vi "CODMn插入数据.vi"(1 "data":T3 {"单位" items=["ug/L", "mg/L", "ppm", "mg/m3", "cm", "ppb", "ug/m3", "%", "nmol/mol", "umol/mol", "MPN/L", "MPN/100ml", "ng/m3", "NTU", "无量纲", "ms/cm", "us/cm"]}, 2 "CODMn关键参数":T2, 3 "SN":string, 5 "table":string, 7 "测量模式":T4(ring)=enum."水样测试", 9 "数据类型":string(combo)="N", 11 "error in (no error)":errorcluster) -> (15 "error out":errorcluster)   [LabVIEW 2016, in "斯坦道CODMn新电路板.lvlib"]
uses:
  <vilib>/Utility/error.llb/DialogType.ctl
panel:
  in  "data 2":T1={"时间"=timestamp(0 s since 1904-01-01), "测量模式"="水样测试", "数据类型"="N", "检测值"=0.0, "单位"="mg/L", "数据标识"="N", "终点滴定数"=0.0, "量程"=0.0, "SN"="", "标样参考值"=0.0, "跨度值"=0.0, "A"=0, "B"=0, "K"=0, "环境温度"=0.0, "加热实时温度"=0.0, "因子编码"="", "X0"=0.0, "X^2"=0.0, "X"=0.0, "B 2"=0.0, "光值1"=0.0, "光值2"=0.0, "光值3"=0.0, "光值4"=0.0, "光值5"=0.0, "光值6"=0.0, "光值7"=0.0, "光值8"=0.0, "测量量程"=0.0, "测量检出限"=0.0, "测量精度"=0.0, "测量间隔"=0.0, "消解温度"=0.0, "消解时长"=0.0, "三项式系数"=0.0, "二次多项式系数"=0.0, "曲线斜率"=0.0, "曲线截距"=0.0, "线性相关系数"=0.0, "空白校准时间"=timestamp(0 s since 1904-01-01), "标样校准时间"=timestamp(0 s since 1904-01-01), "测量信号值"=0.0, "稀释倍数"=0.0, "量程系数"=0.0, "LastTime"=timestamp(0 s since 1904-01-01)}
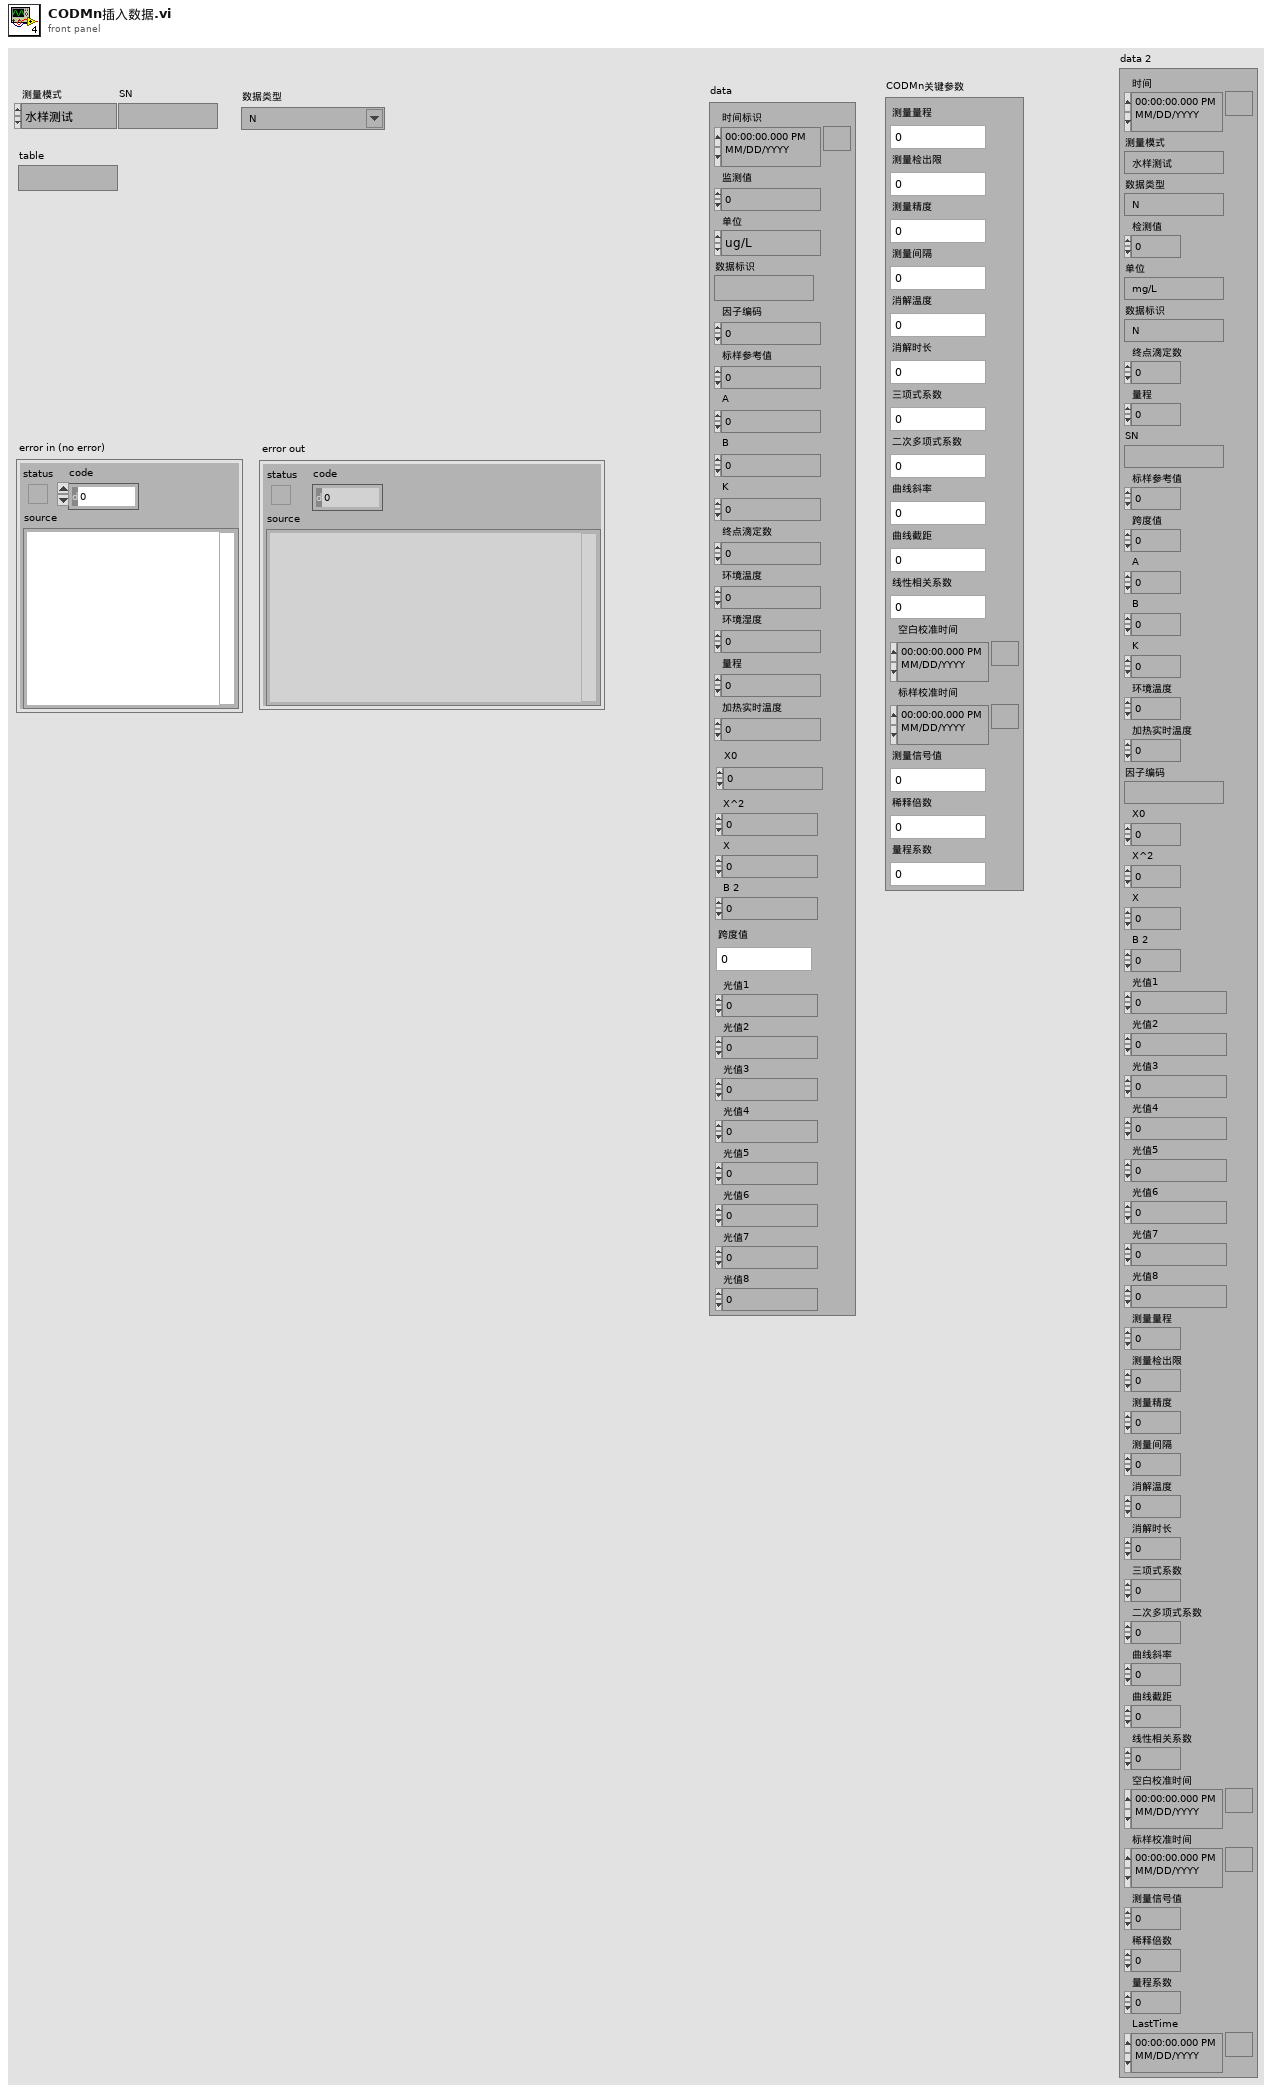
[diagram p1: front panel]
types:
  T1 = cluster{"时间":timestamp, "测量模式":string, "数据类型":string, "检测值":sgl, "单位":string, "数据标识":string, "终点滴定数":sgl, "量程":sgl, "SN":string, "标样参考值":sgl, "跨度值":sgl, "A":u32, "B":u32, "K":u32, "环境温度":sgl, "加热实时温度":sgl, "因子编码":string, "X0":sgl, "X^2":sgl, "X":sgl, "B 2":sgl, "光值1":sgl, "光值2":sgl, "光值3":sgl, "光值4":sgl, "光值5":sgl, "光值6":sgl, "光值7":sgl, "光值8":sgl, "测量量程":sgl, "测量检出限":sgl, "测量精度":sgl, "测量间隔":sgl, "消解温度":sgl, "消解时长":sgl, "三项式系数":sgl, "二次多项式系数":sgl, "曲线斜率":sgl, "曲线截距":sgl, "线性相关系数":sgl, "空白校准时间":timestamp, "标样校准时间":timestamp, "测量信号值":sgl, "稀释倍数":sgl, "量程系数":sgl, "LastTime":timestamp}
  T2 = cluster{"测量量程":sgl, "测量检出限":sgl, "测量精度":sgl, "测量间隔":sgl, "消解温度":sgl, "消解时长":sgl, "三项式系数":sgl, "二次多项式系数":sgl, "曲线斜率":sgl, "曲线截距":sgl, "线性相关系数":sgl, "空白校准时间":timestamp, "标样校准时间":timestamp, "测量信号值":sgl, "稀释倍数":sgl, "量程系数":sgl}
  T3 = cluster{"时间标识":timestamp, "监测值":sgl, "单位":u16, "数据标识":string, "因子编码":u32, "标样参考值":sgl, "A":sgl, "B":sgl, "K":sgl, "终点滴定数":sgl, "环境温度":sgl, "环境湿度":sgl, "量程":sgl, "加热实时温度":sgl, "X0":sgl, "X^2":sgl, "X":sgl, "B 2":sgl, "跨度值":sgl, "光值1":sgl, "光值2":sgl, "光值3":sgl, "光值4":sgl, "光值5":sgl, "光值6":sgl, "光值7":sgl, "光值8":sgl}
  T4 = enum16{"维护数据", "水样测试", "标样核查", "零点核查", "跨度核查", "空白测试", "平行样测试", "加标回收", "空白校准", "标样校准", "初始化（清洗）"}
  T5 = typedef "DialogType.ctl" = u16
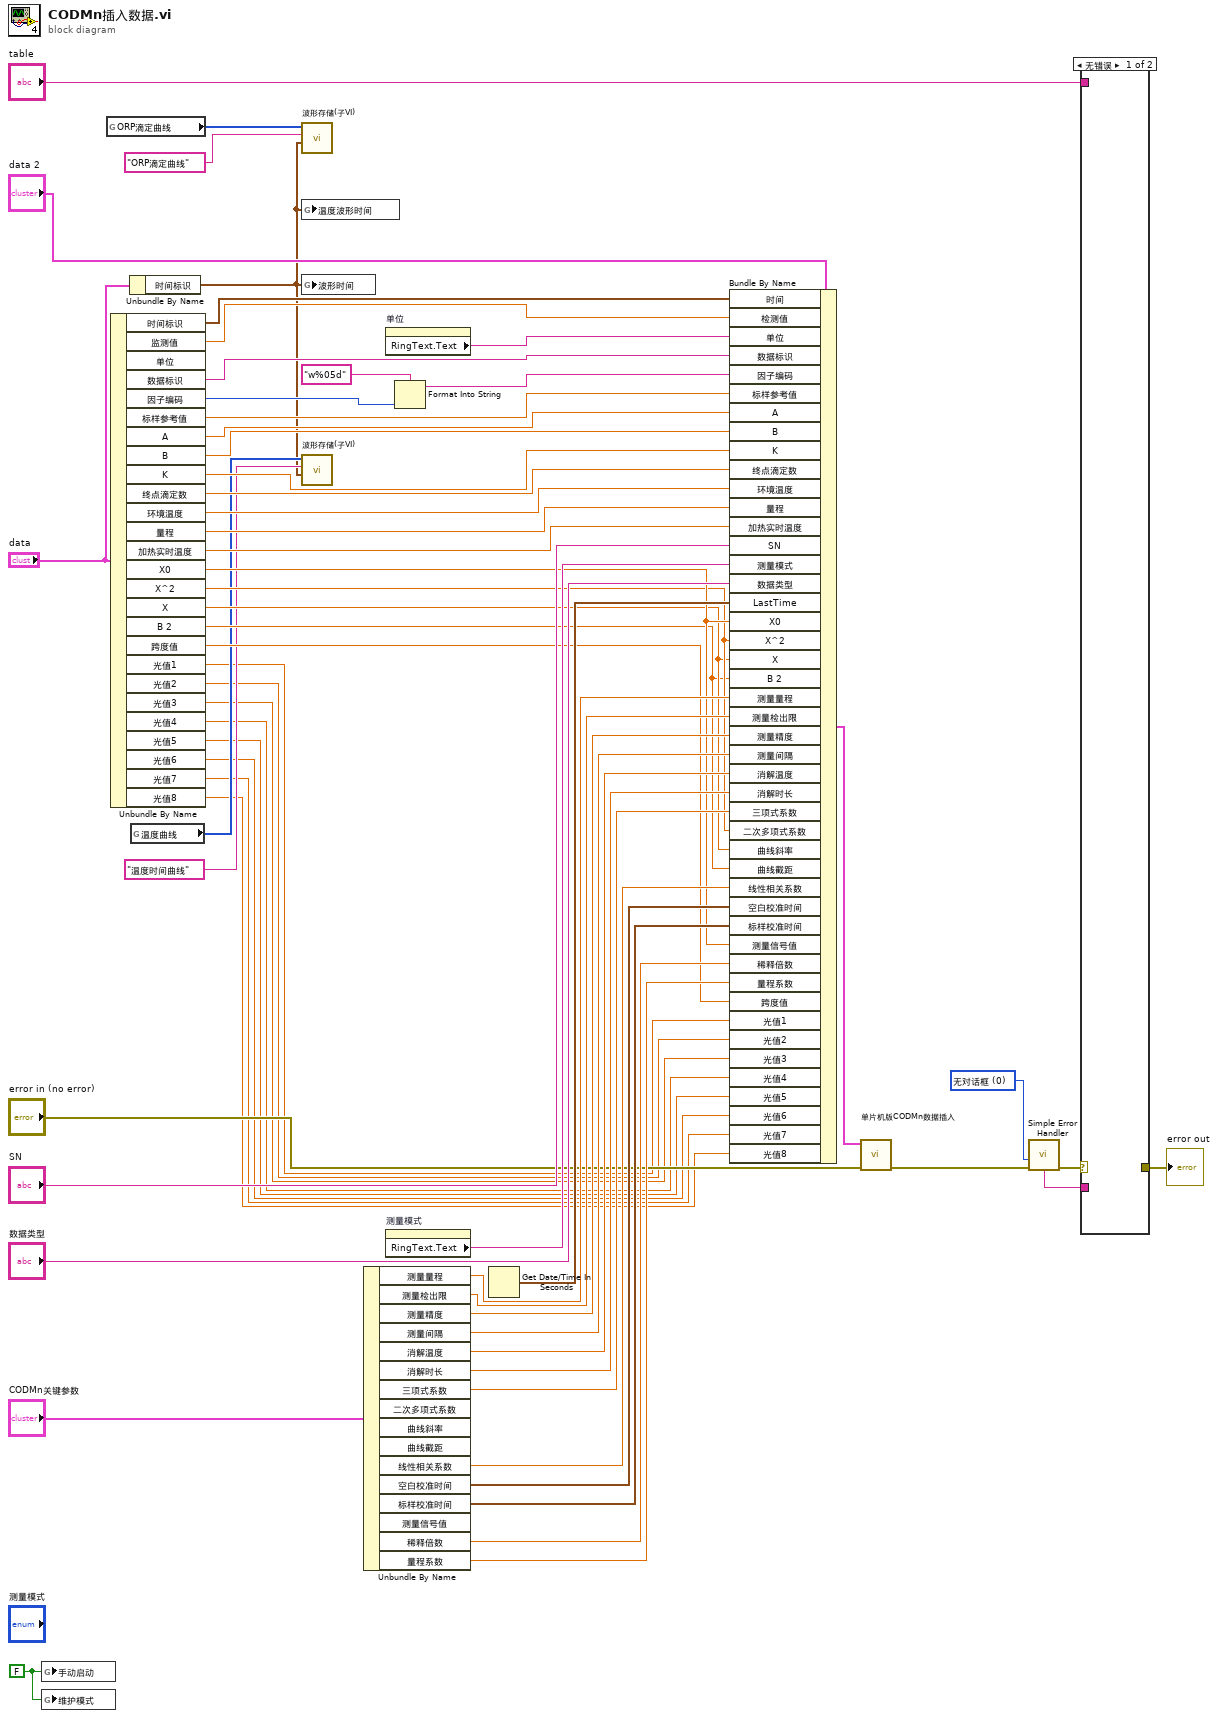
[diagram p0: block diagram]
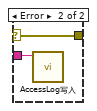
[diagram p2: hidden frame]
diagram:
  w1 = FALSE ("手动启动")
  w61 = T5 0 items=["无对话框", "确定信息", "继续或停止信息", "确定信息＋警告", "继续/停止+警告"] ("type of dialog (OK msg:1)")
  n1 = global write "VARCODMn全局变量.vi" "手动启动"(w1) -> ()
  n2 = global write "VARCODMn全局变量.vi" "维护模式"(w1) -> ()
  n3 = global read "VARCODMn全局变量.vi" "ORP滴定曲线"() -> (w16:u16[])
  n4 = Unbundle By Name("data") -> ("时间标识"=w37:timestamp, "监测值"=w55:sgl, "数据标识"=w53:string, "因子编码"=w51:u32, "标样参考值"=w49:sgl, "A"=w48:sgl, "B"=w47:sgl, "K"=w46:sgl, "终点滴定数"=w45:sgl, "环境温度"=w44:sgl, "量程"=w43:sgl, "加热实时温度"=w42:sgl, "X0"=w26:sgl, "X^2"=w21:sgl, "X"=w20:sgl, "B 2"=w19:sgl, "跨度值"=w22:sgl, "光值1"=w9:sgl, "光值2"=w8:sgl, "光值3"=w7:sgl, "光值4"=w6:sgl, "光值5"=w5:sgl, "光值6"=w4:sgl, "光值7"=w3:sgl, "光值8"=w2:sgl)  [unwired: 1 out]
  n5 = Unbundle By Name("data") -> ("时间标识"=w12:timestamp)
  n6 = global read "VARCODMn全局变量.vi" "温度曲线"() -> (w14:u16[])
  n7 = call "波形存储(子VI).vi"("波形时间"=w12, "condition"="ORP滴定曲线", "ORP滴定曲线"=w16) -> ()  [unwired: 9 in]
  n8 = global write "VARCODMn全局变量.vi" "温度波形时间"(w12) -> ()
  n9 = global write "VARCODMn全局变量.vi" "波形时间"(w12) -> ()
  n10 = call "波形存储(子VI).vi"("波形时间"=w12, "condition"="温度时间曲线", "ORP滴定曲线"=w14) -> ()  [unwired: 9 in]
  n11 = Unbundle By Name("CODMn关键参数") -> ("测量量程"=w36:sgl, "测量检出限"=w35:sgl, "测量精度"=w34:sgl, "测量间隔"=w33:sgl, "消解温度"=w32:sgl, "消解时长"=w31:sgl, "三项式系数"=w30:sgl, "线性相关系数"=w29:sgl, "空白校准时间"=w28:timestamp, "标样校准时间"=w27:timestamp, "稀释倍数"=w25:sgl, "量程系数"=w24:sgl)  [unwired: 4 out]
  n12 = property on="单位" class="Ring (严格)"() -> ("RingText.Text"=w54:string)  [unwired: 2 in, 2 out]
  n13 = property on="测量模式" class="Enum (严格)"() -> ("RingText.Text"=w40:string)  [unwired: 2 in, 2 out]
  n14 = Format Into String(format string="w%05d" ("格式字符串"), w51) -> (resulting string=w50:string)  [unwired: 2 in, 1 out]
  n15 = Get Date/Time In Seconds() -> (seconds since 1Jan1904=w38:timestamp)
  n16 = Bundle By Name(cluster="data 2", "时间"=w37, "检测值"=w55, "单位"=w54, "数据标识"=w53, "因子编码"=w50, "标样参考值"=w49, "A"=w48, "B"=w47, "K"=w46, "终点滴定数"=w45, "环境温度"=w44, "量程"=w43, "加热实时温度"=w42, "SN"="SN", "测量模式"=w40, "数据类型"="数据类型", "LastTime"=w38, "X0"=w26, "X^2"=w21, "X"=w20, "B 2"=w19, "测量量程"=w36, "测量检出限"=w35, "测量精度"=w34, "测量间隔"=w33, "消解温度"=w32, "消解时长"=w31, "三项式系数"=w30, "二次多项式系数"=w21, "曲线斜率"=w20, "曲线截距"=w19, "线性相关系数"=w29, "空白校准时间"=w28, "标样校准时间"=w27, "测量信号值"=w26, "稀释倍数"=w25, "量程系数"=w24, "跨度值"=w22, "光值1"=w9, "光值2"=w8, "光值3"=w7, "光值4"=w6, "光值5"=w5, "光值6"=w4, "光值7"=w3, "光值8"=w2) -> (w17:T1)
  n17 = call "单片机版CODMn数据插入.vi"("data"=w17, "错误输入（无错误）"="error in (no error)") -> ("错误输出"=w11:errorcluster)  [unwired: 8 in]
  n18 = call <vilib>:"Simple Error Handler.vi"("type of dialog (OK msg:1)"=w61, "error in (no error)"=w11) -> ("error out"=w60:errorcluster, "message"=w59:string)  [unwired: 3 in, 3 out]
  n19 = case shown="无错误" w60 {
    selector: w60 -> [_ w62]
    tunnel: w59 -> [_ w63]
    tunnel: [_ w62] -> w58
    tunnel: "table" -> [_ _]
    frame No Error {
    }
    frame Error {
      n20 = call "AccessLog写入.vi"("Log"=w63) -> ()  [unwired: 11 in]
    }
  }
  "error out" <- w58
